vi "GetDBPath.vi"() -> (0 "Connection":string)   [LabVIEW 2014, in "DataBase.lvlib"]
uses:
  DataBase.lvlib
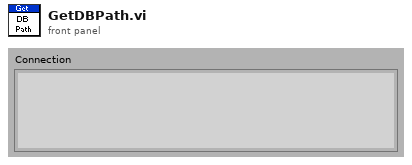
[diagram p1: front panel]
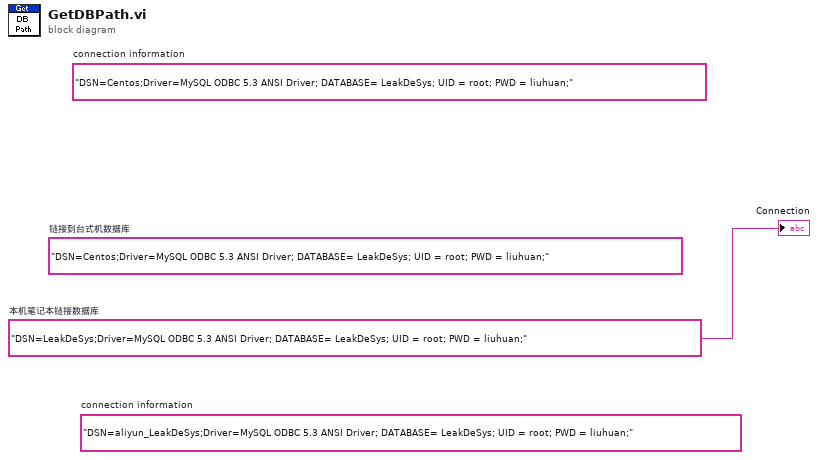
[diagram p0: block diagram]
diagram:
  (unwired) "DSN=aliyun_LeakDeSys;Driver=MySQL ODBC 5.3 ANSI Driver; DATABASE= LeakDeSys; UID = root; PWD = liuhuan;"  # connection information
  (unwired) "DSN=Centos;Driver=MySQL ODBC 5.3 ANSI Driver; DATABASE= LeakDeSys; UID = root; PWD = liuhuan;"  # connection information
  w1 = "DSN=LeakDeSys;Driver=MySQL ODBC 5.3 ANSI Driver; DATABASE= LeakDeSys; UID = root; PWD = liuhuan;"  # 本机笔记本链接数据库
  (unwired) "DSN=Centos;Driver=MySQL ODBC 5.3 ANSI Driver; DATABASE= LeakDeSys; UID = root; PWD = liuhuan;"  # 链接到台式机数据库
  "Connection" <- w1
